vi "Send Files to PXI.vi"() -> ()   [LabVIEW 2013]
doc: "This VI sends all the files in the Host PC located at \"mf3_labview\\Configuration Files\" to the PXI.\n\nYou just need to run it!"
uses:
  <vilib>/FTP/NI_FTP.lvlib
panel:
  in  "Destination":string="C:\\ni-rt\\fsuarez"
  out "error out":errorcluster
  in  "PXI IP":string="192.168.0.5"
  # "This VI sends all the files in the Host PC located at \n\"mf3_labview/Configuration Files\" to the PXI.\n\nYou just need to run it!"
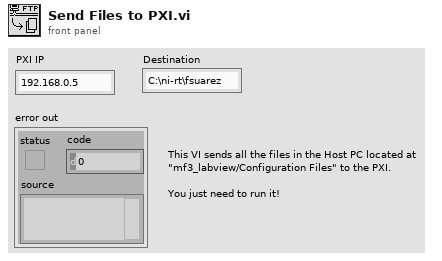
[diagram p1: front panel]
types:
  T1 = typedef "NI_FTP.lvlib/FTP Session.ctl" = refnum<k5>
  T2 = cluster{"remote path":string, "local path":path, "binary":bool, "data":string}
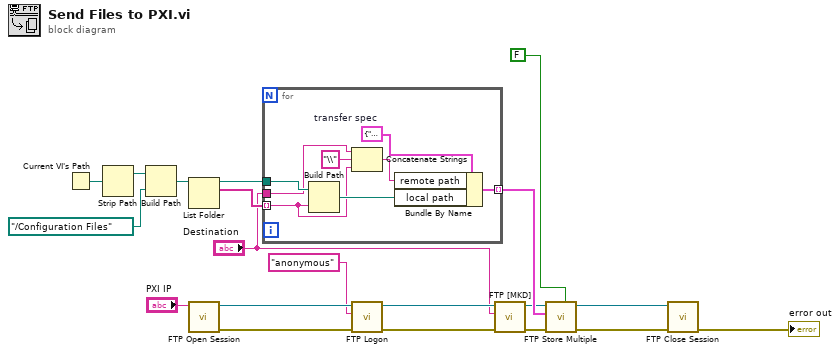
[diagram p0: block diagram]
diagram:
  n1 = Current VI's Path() -> (path=w15:path)
  n2 = Strip Path(path=w15) -> (stripped path=w14:path)  [unwired: 1 out]
  n3 = Build Path(base path=w14, name or relative path=path "../Configuration Files" ("Relative Path to be Sent")) -> (appended path=w13:path)
  n4 = List Folder(path=w13) -> (path out=w12:path, filenames=w11:string[])  [unwired: 3 in, 2 out]
  n5 = call <vilib>:"FTP Open Session.vi"("address"="PXI IP") -> ("error out"=w17:errorcluster, "ftp session"=w20:T1)  [unwired: 7 in, 2 out]
  n6 = for {
    tunnel: w12 -> [w28]
    tunnel: w11 -> [w22] mode=indexing
    tunnel: [w25] -> w8 mode=indexing
    tunnel: "Destination" -> [w23]
    w27 = T2 {"remote path"="", "local path"=path "", "binary"=FALSE, "data"=""}  # transfer spec
    n7 = Build Path(base path=w28, name or relative path=w22) -> (appended path=w24:path)
    n8 = Concatenate Strings(w23, "\\" ("user"), w22) -> (w26:string)
    n9 = Bundle By Name(cluster=w27, "remote path"=w26, "local path"=w24) -> (w25:T2)
  }
  n10 = call <vilib>:"FTP Logon.vi"("error in (no error)"=w17, "user"="anonymous", "ftp session"=w20) -> ("error out"=w4:errorcluster, "ftp session out"=w5:T1)  [unwired: 5 in, 2 out]
  n11 = call <vilib>:"FTP [MKD].vi"("error in (no error)"=w4, "directory path"="Destination", "ftp session"=w5) -> ("error out"=w1:errorcluster, "ftp session out"=w2:T1)  [unwired: 5 in, 2 out]
  n12 = call <vilib>:"FTP Store Multiple.vi"("active (T)"=FALSE, "error in (no error)"=w1, "file specifications"=w8, "ftp session"=w2) -> ("error out"=w9:errorcluster, "ftp session out"=w10:T1)  [unwired: 5 in, 1 out]
  n13 = call <vilib>:"FTP Close Session.vi"("error in (no error)"=w9, "ftp session"=w10) -> ("error out"=→"error out":errorcluster)  [unwired: 6 in, 3 out]
